vi "parseDataOccu.vi"(0 "array":u8[](array[numeric])) -> (1 "Event (1 bytes)":u16, 2 "TS (4  bytes)":u32)   [LabVIEW 2011]
panel:
  out "input data size (in bytes)":i32
  out "input data (in hex)":string[](array[string])
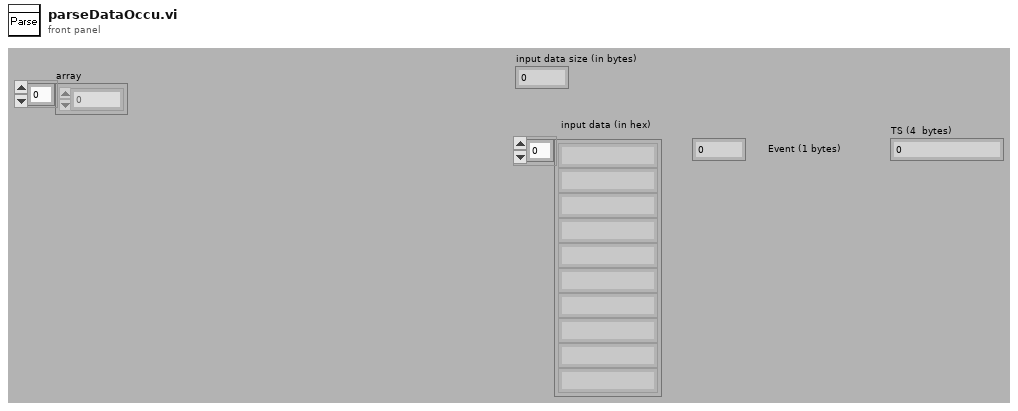
[diagram p1: front panel]
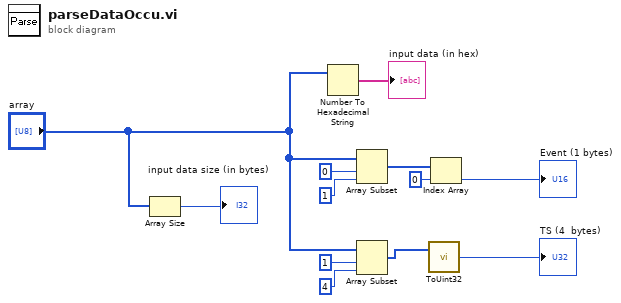
[diagram p0: block diagram]
diagram:
  n1 = Array Size(array="array") -> (size(s)=→"input data size (in bytes)":i32)
  n2 = Number To Hexadecimal String(2:"array") -> (0:→"input data (in hex)":string[])  [unwired: 1 in]
  n3 = Array Subset(array="array", index=0 ("x"), length=1 ("x")) -> (w10:u8[])
  n4 = Array Subset(array="array", index=1 ("x"), length=4 ("x")) -> (w3:u8[])
  n5 = call "ToUint32.vi"("array"=w3) -> ("sp float"=→"TS (4  bytes)":u32)  [unwired: 1 in]
  n6 = Index Array(array=w10, index=0) -> (element=→"Event (1 bytes)":u8)
